vi "DFD Get MRate CIC Parameters.vi"(8 "error in (no error)":errorcluster, 11 "multirate filter in":T3={"mMRate_Structure"=enum."IIR", "mMRate_Mode"=0, "mMRate_Factor"=-1, "mMRate_FIRParams"={"mMRate_FIR_H"=[], "mMRate_FIR_IsNyquist?"=FALSE, "mMRate_FIR_IsSymmetric?"=FALSE}, "mMRate_CICParams"={"mMRate_CIC_#Stage"=0, "mMRate_CIC_Lag"=0, "mMRate_CIC_Type"=enum."Lowpass"}, "mMRate_Order"=0, "mMRate_Version"="2.0", "mMRate_Comments"="", "mMRate_RationalFactor"={"mMRate_L"=-1, "mMRate_M"=-1}, "mMRate_Fs"=1.0, "mMRate_Quantized?"=FALSE, "mMRate_QFilterGain"=1.0, "mMRate_CoefWl"=16, "mMRate_Scaling"={"mMRate_ScaleByPowerOf2?"=FALSE, "mMRate_ScaleType"=enum."No Norm"}, "mMRate_InputWl"=16, "mMRate_OutputWl"=16, "mMRate_OutputMode"=enum."Truncation", "mMRate_MultMode"=enum."Truncated", "mMRate_BitPruning"=FALSE, "mMRate_GainWl"=16, "mMRate_OutputFwl"=0, "mMRate_SumIwl"=0, "mMRate_InputIwl "=16, "mMRate_SumWl"=32, "mMRate_CoefIwl"=0} {"mMRate_SumWl" min=1 max=32 step=1; "mMRate_InputIwl" min=1 max=32 step=1; "mMRate_GainWl" min=1 max=32 step=1; "mMRate_OutputWl" min=1 max=32 step=1; "mMRate_InputWl" min=1 max=32 step=1; "mMRate_CoefWl" min=1 max=32 step=1; "mMRate_Mode" items=["Default"=-1, "No Rate Change"=0, "Interpolation"=1, "Decimation"=2, "Interpolated"=3, "Rational"=4]}) -> (0 "error out":errorcluster, 1 "filtering mode":T2=2 items=["No Rate Change", "Interpolation", "Decimation"], 2 "factor":i32, 3 "CIC parameters":T1, 5 "h(n)":dbl[](array[numeric]))   [LabVIEW 2017, in "NI_DigFilterLicensed.lvlib"]
doc: "Retrieves the transfer function coefficients, sampling frequency conversion factor, filtering mode, and filter parameters of a cascaded integrator comb (CIC) filter."
uses:
  <vilib>/addons/Digital Filter Design/NI_DigFilterLicensed.lvlib
  <vilib>/addons/Digital Filter Design/_Objects.llb/DFD Multirate Filter Obj.ctl
  <vilib>/addons/Digital Filter Design/_Objects.llb/DFD Multirate Mode.ctl
  <vilib>/addons/Digital Filter Design/_Objects.llb/DFD Coef Norm Type.ctl
  <vilib>/addons/Digital Filter Design/_Objects.llb/DFD Round-off Mode.ctl
  <vilib>/addons/Digital Filter Design/_Objects.llb/DFD FXP MRate Multiply Mode.ctl
  <vilib>/addons/Digital Filter Design/_Objects.llb/DFD Multirate Filtering Mode.ctl
  <vilib>/addons/Digital Filter Design/_Misc.llb/dfd_Error Handlers (Single).vi
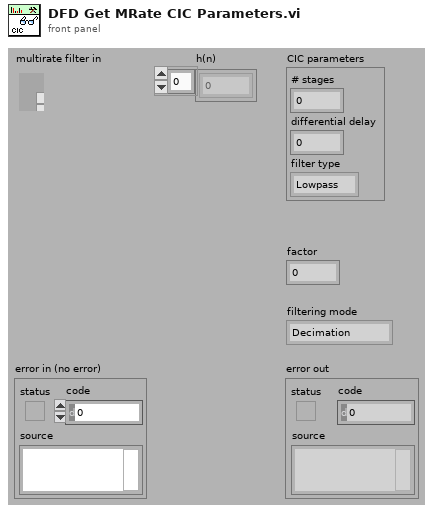
[diagram p1: front panel]
types:
  T1 = cluster{"# stages":i32, "differential delay":i32, "filter type":enum16{"Lowpass", "Highpass"}}
  T2 = typedef "NI_DigFilterLicensed.lvlib/DFD Multirate Filtering Mode.ctl" = u16
  T3 = typedef "NI_DigFilterLicensed.lvlib/DFD Multirate Filter Obj.ctl" = cluster{"mMRate_Structure":enum16{"CIC", "FIR", "IIR", "Lattice"}, "mMRate_Mode":T4, "mMRate_Factor":i32, "mMRate_FIRParams":cluster{"mMRate_FIR_H":dbl[], "mMRate_FIR_IsNyquist?":bool, "mMRate_FIR_IsSymmetric?":bool}, "mMRate_CICParams":cluster{"mMRate_CIC_#Stage":i32, "mMRate_CIC_Lag":i32, "mMRate_CIC_Type":enum16{"Lowpass", "Highpass"}}, "mMRate_Order":i32, "mMRate_Version":string, "mMRate_Comments":string, "mMRate_RationalFactor":cluster{"mMRate_L":i32, "mMRate_M":i32}, "mMRate_Fs":dbl, "mMRate_Quantized?":bool, "mMRate_QFilterGain":dbl, "mMRate_CoefWl":i16, "mMRate_Scaling":cluster{"mMRate_ScaleByPowerOf2?":bool, "mMRate_ScaleType":T5}, "mMRate_InputWl":i16, "mMRate_OutputWl":i16, "mMRate_OutputMode":T6, "mMRate_MultMode":T7, "mMRate_BitPruning":bool, "mMRate_GainWl":i16, "mMRate_OutputFwl":i16, "mMRate_SumIwl":i16, "mMRate_InputIwl ":i16, "mMRate_SumWl":i16, "mMRate_CoefIwl":i16}
  T4 = typedef "NI_DigFilterLicensed.lvlib/DFD Multirate Mode.ctl" = i16
  T5 = typedef "NI_DigFilterLicensed.lvlib/DFD Coef Norm Type.ctl" = enum16{"No Norm", "Time Domain 1-Norm", "Time Domain 2-Norm", "Time Domain Inf-Norm"}
  T6 = typedef "NI_DigFilterLicensed.lvlib/DFD Round-off Mode.ctl" = enum16{"Nearest", "Truncation"}
  T7 = typedef "NI_DigFilterLicensed.lvlib/DFD FXP MRate Multiply Mode.ctl" = enum16{"Truncated", "Full"}
  T8 = cluster{"num of stages":i32, "lag":i32, "type":enum16{"Lowpass", "Highpass"}}
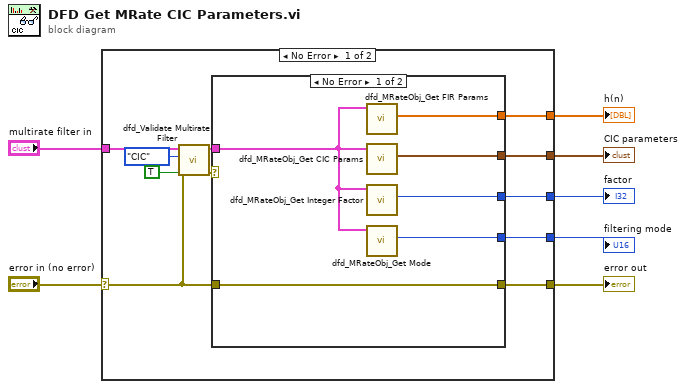
[diagram p0: block diagram]
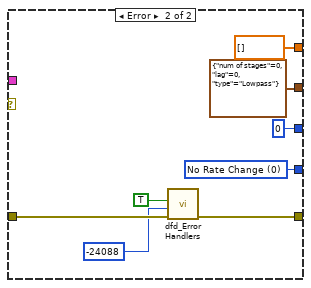
[diagram p2: hidden frame]
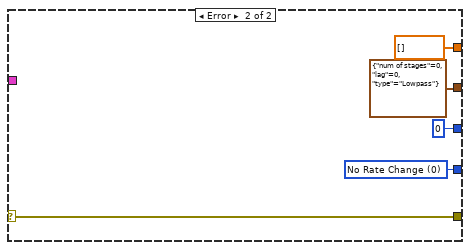
[diagram p3: hidden frame]
diagram:
  n1 = case shown="No Error" "error in (no error)" {
    selector: "error in (no error)" -> [w10 w33]
    tunnel: "multirate filter in" -> [w17 _]
    tunnel: [w14 dbl[] [] ("h(n)")] -> w2
    tunnel: [w13 T8 {"num of stages"=0, "lag"=0, "type"=enum."Lowpass"} ("CIC params")] -> w5
    tunnel: [w12 0 ("factor")] -> w3
    tunnel: [w11 w34] -> w4
    tunnel: [w9 w33] -> w1
    frame No Error {
      n2 = call <vilib>:"dfd_Validate Multirate Filter.vi"("error in (no error)"=w10, "skip FXP? (T)"=TRUE, "preferred structure"=enum16{"CIC", "FIR", "IIR", "Lattice"}."CIC" ("prefered structure"), "multirate filter in"=w17) -> ("error out"=w16:errorcluster, "multirate filter out"=w15:T3)  [unwired: 6 out]
      n3 = case shown="No Error" w16 {
        tunnel: w15 -> [w24 _]
        tunnel: [w23 dbl[] [] ("h(n)")] -> w14
        tunnel: [w22 T8 {"num of stages"=0, "lag"=0, "type"=enum."Lowpass"} ("CIC params")] -> w13
        tunnel: [w21 0 ("factor")] -> w12
        tunnel: [w20 w30] -> w11
        tunnel: w10 -> [w19 w28]
        tunnel: [w19 w25] -> w9
        frame No Error {
          n4 = call <vilib>:"dfd_MRateObj_Get FIR Params.vi"("multirate filter in"=w24) -> ("h(n)"=w23:dbl[])  [unwired: 10 out]
          n5 = call <vilib>:"dfd_MRateObj_Get CIC Params.vi"("multirate filter in"=w24) -> ("CIC params"=w22:T8)  [unwired: 10 out]
          n6 = call <vilib>:"dfd_MRateObj_Get Integer Factor.vi"("multirate filter in"=w24) -> ("factor"=w21:i32)  [unwired: 10 out]
          n7 = call <vilib>:"dfd_MRateObj_Get Mode.vi"("multirate filter in"=w24) -> ("mode"=w20:T4)  [unwired: 10 out]
        }
        frame Error {
          w30 = T4 0 items=["Default"=-1, "No Rate Change"=0, "Interpolation"=1, "Decimation"=2, "Interpolated"=3, "Rational"=4] ("mode")
          n8 = call-poly <vilib>:"dfd_Error Handlers.vi"("error in (no error)"=w28, "error code"=-24088 ("ERR_CIC_EXPECTED"), "condition failed?"=TRUE) -> ("error out"=w25:errorcluster)  [unwired: 8 out]
        }
      }
    }
    frame Error {
      w34 = T4 0 items=["Default"=-1, "No Rate Change"=0, "Interpolation"=1, "Decimation"=2, "Interpolated"=3, "Rational"=4] ("mode")
    }
  }
  "filtering mode" <- w4
  "error out" <- w1
  "h(n)" <- w2
  "factor" <- w3
  "CIC parameters" <- w5
